vi "Get Auth Details for NI Web Server.vi"(0 "LabVIEW Web Service Request":refnum<class "Web Request.lvclass">, 11 "error in (no error)":errorcluster) -> (4 "LabVIEW Web Service Request out":refnum<class "Web Request.lvclass">, 6 "user ID":string, 8 "username":string, 10 "privileges":string[](array[string]), 15 "error out":errorcluster)   [LabVIEW 2020, in "NI_WebServices.lvlib" / "Web Request.lvclass"]
doc: "Returns the authentication details associated with the current HTTP request. The authentication details indicate which user account is logged in to the NI Web Server."
uses:
  <vilib>/wsapi/Web Request.lvclass
  <vilib>/wsapi/Web Request.lvclass/Web Request.ctl
  <vilib>/wsapi/NI_WebServices.lvlib
  ws_runtime.dll
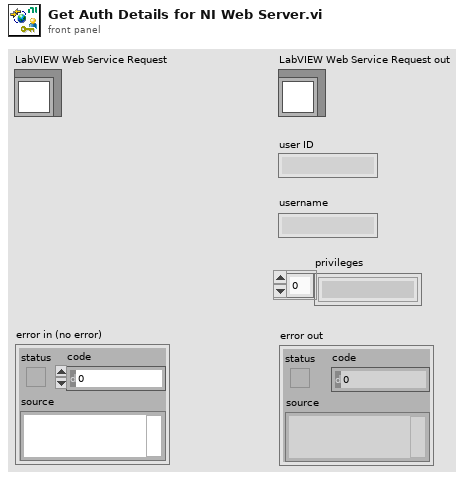
[diagram p1: front panel]
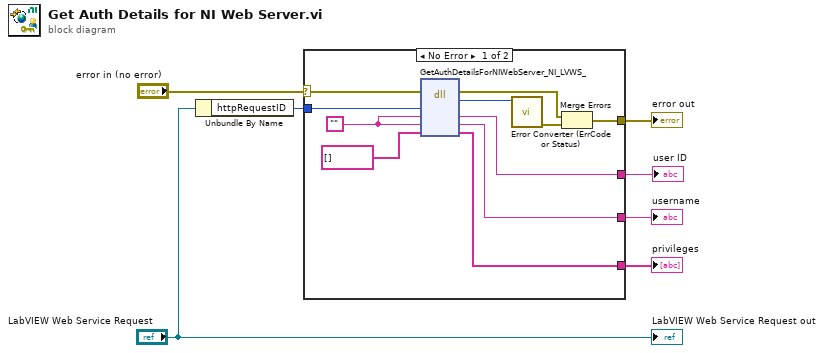
[diagram p0: block diagram]
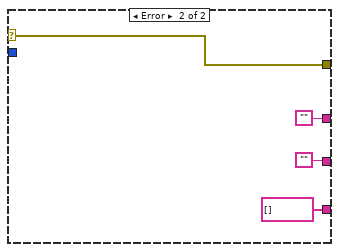
[diagram p2: hidden frame]
diagram:
  n1 = Unbundle By Name("LabVIEW Web Service Request") -> ("httpRequestID"=w3:u32)
  n2 = case shown="No Error" "error in (no error)" {
    selector: "error in (no error)" -> [w10 w22]
    tunnel: [w18 ""] -> w7
    tunnel: [w17 string[] []] -> w6
    tunnel: [w15 w22] -> w5
    tunnel: w3 -> [w14 _]
    tunnel: [w9 ""] -> w1
    frame No Error {
      w8 = ""
      n3 = dll-call lib="ws_runtime.*" fn="GetAuthDetailsForNIWebServer_NI_LVWS_"(error in=w10, "httpRequestID"=w14, "userID"=w8, "username"=w8, "privileges"=string[] [] ("groups")) -> (error out=w16:errorcluster, "return type"=w13:i32, "userID"=w9:string, "username"=w18:string, "privileges"=w17:string[])  [unwired: 3 in, 1 out]
      n4 = call <vilib>:"Error Converter (ErrCode or Status).vi"("error code"=w13) -> ("error out"=w12:errorcluster)  [unwired: 10 in]
      n5 = Merge Errors(w16, w12) -> (w15:errorcluster)
    }
    frame Error {
    }
  }
  "error out" <- w5
  "username" <- w7
  "privileges" <- w6
  "user ID" <- w1
  "LabVIEW Web Service Request out" <- "LabVIEW Web Service Request"
